vi "QPD2.vi"() -> ()   [LabVIEW 2019]
uses:
  <vilib>/DAQmx/read.llb/DAQmx Read (Analog 1D Wfm NChan NSamp).vi
  <vilib>/DAQmx/miscellaneous.llb/DAQmx Fill In Error Info.vi
panel:
  in  "Tab Control":T1(tab)
  out "Waveform Chart":waveform(dbl)[](graph)
  in  "Frequency":dbl=1.0
  in  "Amplitude":dbl=1.0
  in  "Duration":dbl=1.0
  in  "stop 2":bool caption="stop"
  in  "Start Signal Gen":bool
  in  "Stop Signal Gen":bool
  out "QPD XY 2":cluster{"Array":dbl[], "Array":dbl[]}(graph)
  out "error out 2":errorcluster
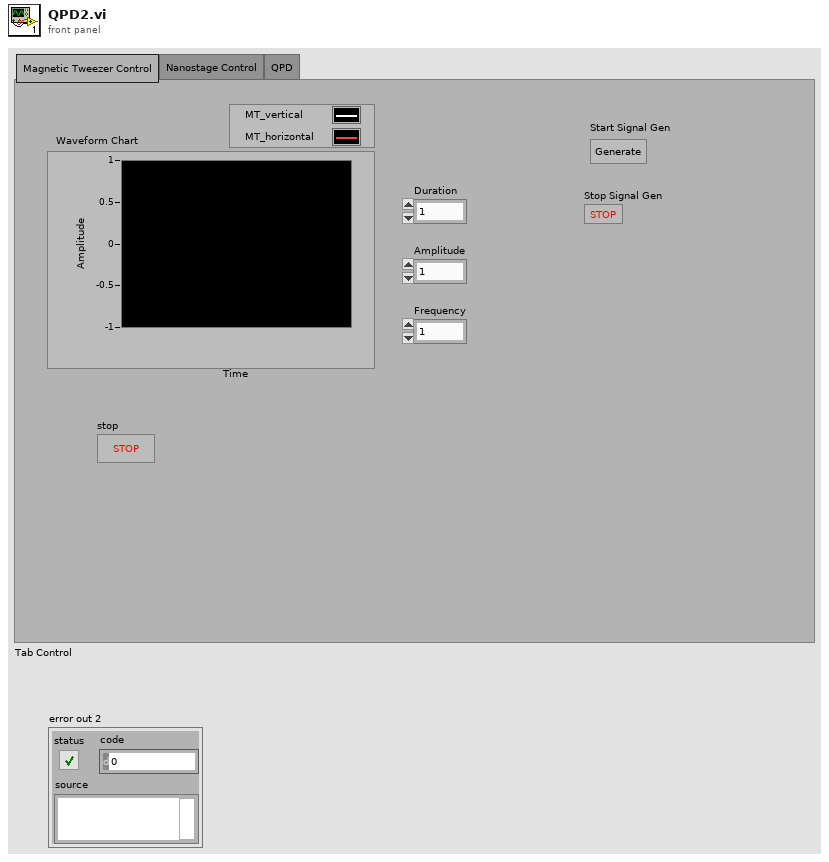
[diagram p1: front panel]
types:
  T1 = enum32{"Magnetic Tweezer Control", "Nanostage Control", "QPD"}
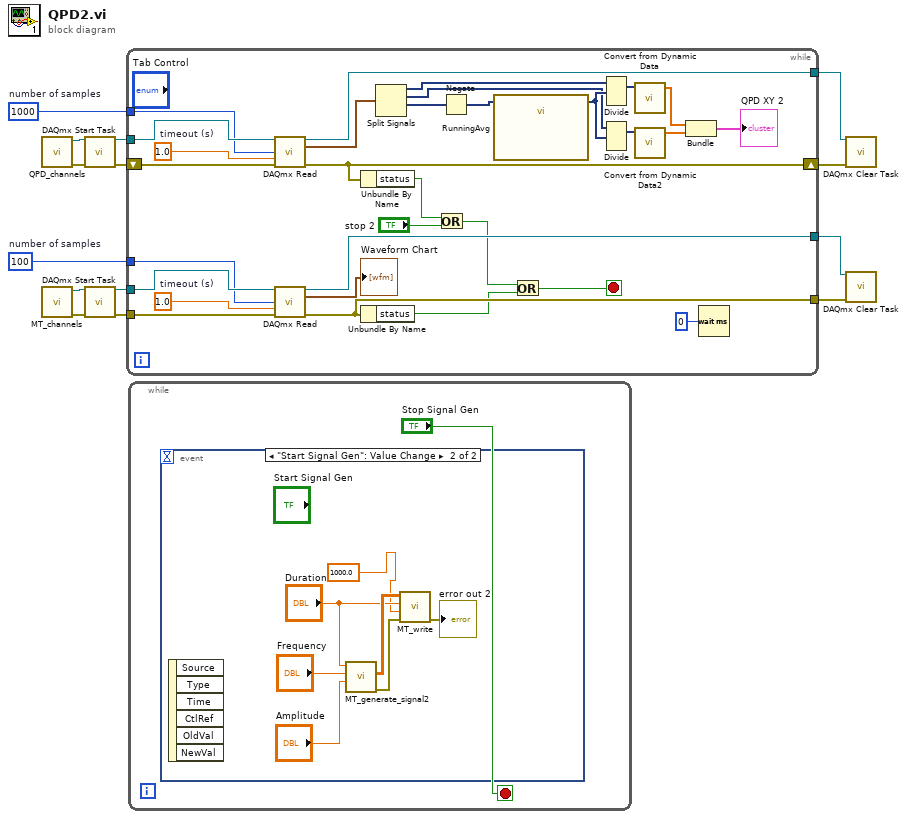
[diagram p0: block diagram]
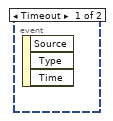
[diagram p2: hidden frame]
diagram:
  w7 = 100  # number of samples
  w12 = 1000  # number of samples
  n1 = call "QPD_channels.vi"() -> ("error out"=w2:errorcluster, "task out"=w1:refnum<k21>)  [unwired: 10 in]
  n2 = call "MT_channels.vi"() -> ("error out"=w3:errorcluster, "task out"=w4:refnum<k21>)  [unwired: 10 in]
  n3 = call <vilib>:"DAQmx Start Task.vi"("task/channels in"=w1, "error in"=w2) -> ("task out"=w14:refnum<k21>, "error out"=w13:errorcluster)  [unwired: 12 in]
  n4 = call <vilib>:"DAQmx Start Task.vi"("task/channels in"=w4, "error in"=w3) -> ("task out"=w9:refnum<k21>, "error out"=w8:errorcluster)  [unwired: 12 in]
  n5 = while {
    tunnel: w14 -> [w44]
    tunnel: w12 -> [w41]
    tunnel: [w42] -> w10
    shift-right: [w39] -> w11
    shift-left: w13 -> [w43]
    tunnel: w9 -> [w24]
    tunnel: w8 -> [w23]
    tunnel: w7 -> [w22]
    tunnel: [w21] -> w6
    tunnel: [w20] -> w5
    stop <- w18 stop-if-true
    w25 = 1.0  # timeout (s)
    w37 = 1.0  # timeout (s)
    n6 = call-poly <vilib>:"DAQmx Read.vi"("task/channels in"=w44, "number of samples per channel"=w41, "timeout"=w37, "error in"=w43) -> ("task out"=w42:refnum<k21>, "data"=w29:waveform(dbl)[], "error out"=w39:errorcluster)  [unwired: 9 in]
    n7 = call-poly <vilib>:"DAQmx Read.vi"("task/channels in"=w24, "number of samples per channel"=w22, "timeout"=w25, "error in"=w23) -> ("task out"=w21:refnum<k21>, "data"=→"Waveform Chart":waveform(dbl)[], "error out"=w20:errorcluster)  [unwired: 9 in]
    n8 = Unbundle By Name(w39) -> ("status"=w40:bool)
    n9 = Unbundle By Name(w20) -> ("status"=w16:bool)
    n10 = Split Signals(w29) -> (w28:dynamicdata, w27:dynamicdata, w26:dynamicdata)  [unwired: 4 in, 1 out]
    n11 = Or(x=w40, y="stop 2") -> (x .or. y?=w17:bool)
    n12 = Negate(x=w26) -> (-x=w36:dynamicdata)
    n13 = call "RunningAvg"("Signal"=w36) -> ("Filtered Signal"=w30:dynamicdata)  [unwired: 9 in, 1 out]
    n14 = Or(x=w17, y=w16) -> (x .or. y?=w18:bool)
    n15 = Divide(1:w30, 2:w28) -> (0:w35:dynamicdata)  [unwired: 1 in, 1 out]
    n16 = Divide(1:w30, 2:w27) -> (0:w34:dynamicdata)  [unwired: 1 in, 1 out]
    n17 = call "Convert from Dynamic Data"("Dynamic Data Type"=w35) -> ("Array"=w33:dbl[])  [unwired: 3 in]
    n18 = call "Convert from Dynamic Data2"("Dynamic Data Type"=w34) -> ("Array"=w32:dbl[])  [unwired: 3 in]
    n19 = Bundle("Array"=w33, "Array"=w32) -> (→"QPD XY 2":cluster{"Array":dbl[], "Array":dbl[]})  [unwired: 1 in]
    n20 = Wait (ms)(milliseconds to wait=u32 0) -> ()  [unwired: 1 out]
  }
  n21 = while {
    stop <- "Stop Signal Gen" stop-if-true
    n22 = event shown="[1] \"Start Signal Gen\": Value Change" {
      selector: _ -> [_ _]
      dyn-events: _ -> [_ _]
      timeout: _ -> [_ _]
      event Timeout {
        n23 = event-data() -> ()  [unwired: 1 in, 3 out]
      }
      event "Start Signal Gen": Value Change {
        n24 = event-data() -> ()  [unwired: 1 in, 6 out]
        n25 = call "MT_generate_signal2.vi"("Amplitude"="Amplitude", "Frequency"="Frequency", "Duration"="Duration") -> ("error out"=w52:errorcluster, "Signals out"=w51:dbl[][])  [unwired: 6 in, 1 out]
        n26 = call "MT_write.vi"("error in"=w52, "sampling rate"=1000.0, "duration"="Duration", "data"=w51) -> ("error out"=→"error out 2":errorcluster)  [unwired: 7 in]
      }
    }
  }
  n27 = call <vilib>:"DAQmx Clear Task.vi"("task in"=w10, "error in"=w11) -> ()  [unwired: 13 in, 1 out]
  n28 = call <vilib>:"DAQmx Clear Task.vi"("task in"=w6, "error in"=w5) -> ()  [unwired: 13 in, 1 out]
